vi "WS1050_Data Trans.vi"(8 "error in (no error)":errorcluster, 10 "Array 2":string[][](array[string])) -> (0 "error out":errorcluster, 2 "output array":string[](array[string]))   [LabVIEW 2017]
panel:
  out "subarray":string[](array[string])
  out "subarray 4":string[](array[string])
  out "subarray 3":string[](array[string])
  out "subarray 2":string[](array[string])
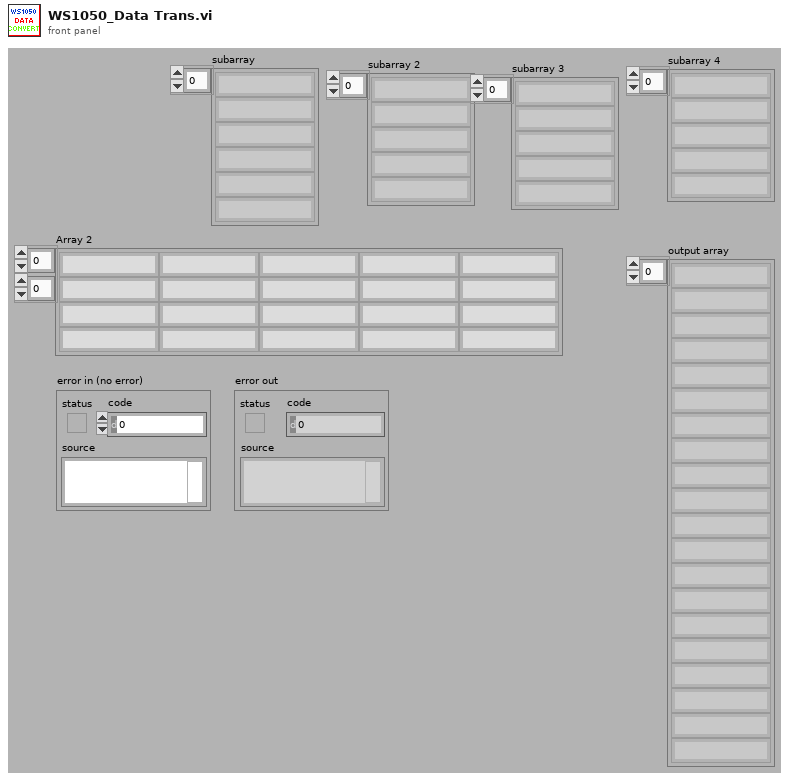
[diagram p1: front panel]
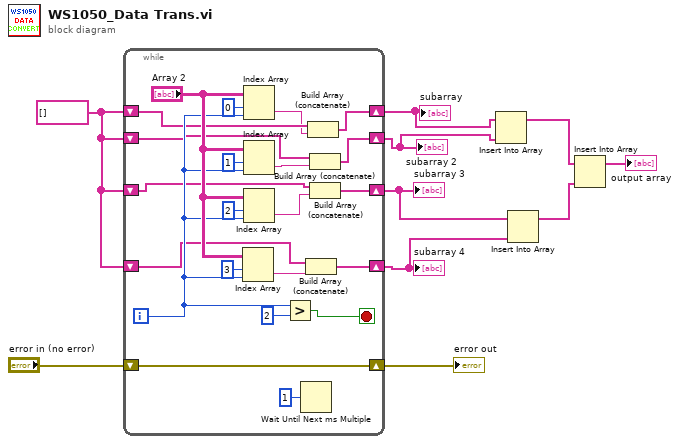
[diagram p0: block diagram]
diagram:
  w10 = string[] []
  n1 = while {
    shift-right: [w23] -> w9
    shift-left: w10 -> [w24]
    shift-right: [w20] -> w7
    shift-left: w10 -> [w19]
    shift-right: [w16] -> w8
    shift-left: w10 -> [w17]
    shift-right: [w13] -> w6
    shift-left: w10 -> [w14]
    shift-right: [w12] -> w1
    shift-left: "error in (no error)" -> [w12]
    i -> [w29]
    stop <- w31 stop-if-true
    n2 = Index Array(array="Array 2", index (row)=3 ("disabled index (row)"), index (col)=w29) -> (element=w15:string)
    n3 = Index Array(array="Array 2", index (row)=0 ("disabled index (row)"), index (col)=w29) -> (element=w22:string)
    n4 = Index Array(array="Array 2", index (row)=1 ("disabled index (row)"), index (col)=w29) -> (element=w18:string)
    n5 = Index Array(array="Array 2", index (row)=2 ("disabled index (row)"), index (col)=w29) -> (element=w21:string)
    n6 = Greater?(x=w29, y=2) -> (0:w31:bool)
    n7 = Wait Until Next ms Multiple(millisecond multiple=u32 1) -> ()  [unwired: 1 out]
    n8 = Build Array (concatenate)(w14, w15) -> (w13:string[])
    n9 = Build Array (concatenate)(w24, w22) -> (w23:string[])
    n10 = Build Array (concatenate)(w17, w18) -> (w16:string[])
    n11 = Build Array (concatenate)(w19, w21) -> (w20:string[])
  }
  "subarray" <- w9
  "subarray 2" <- w8
  "subarray 3" <- w7
  "subarray 4" <- w6
  "error out" <- w1
  n12 = Insert Into Array(array=w9, new element=w8) -> (w5:string[])  [unwired: 1 in]
  n13 = Insert Into Array(array=w7, new element=w6) -> (w4:string[])  [unwired: 1 in]
  n14 = Insert Into Array(array=w5, new element=w4) -> (→"output array":string[])  [unwired: 1 in]
